vi "Circular Buffer Waveform.vi"(6 "Action":T1, 8 "Error In":errorcluster, 9 "New Data":waveform(dbl), 10 "Size":i32) -> (0 "Error Out":errorcluster, 1 "Buffer Out":waveform(dbl)[](array[waveform]), 2 "Iterations":i32, 5 "Ready":bool)   [LabVIEW 2015]
uses:
  Circular Buffer Operations.ctl
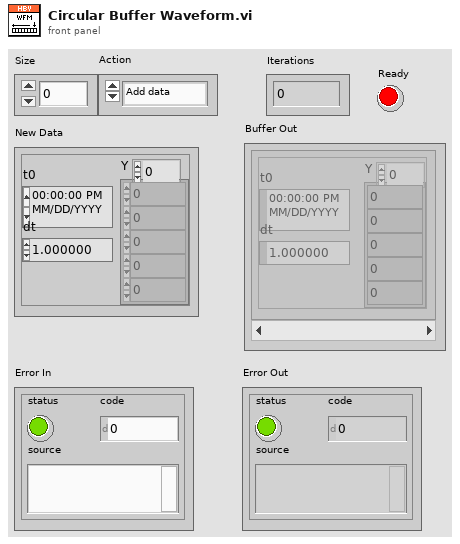
[diagram p1: front panel]
types:
  T1 = typedef "Circular Buffer Operations.ctl" = enum16{"Add data", "Reset"}
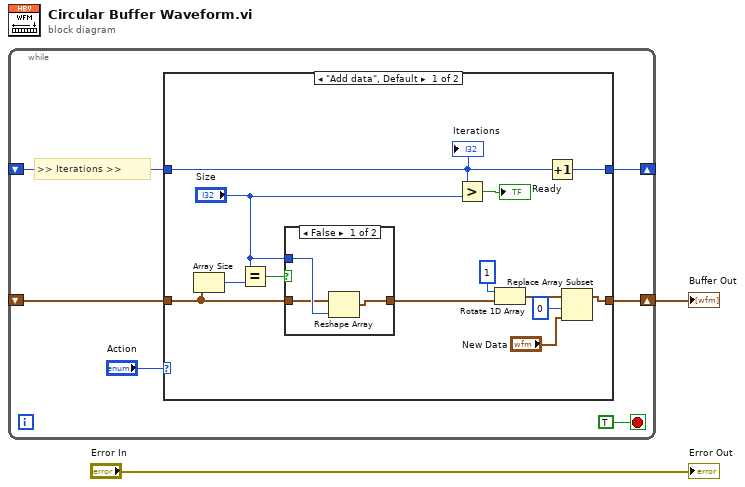
[diagram p0: block diagram]
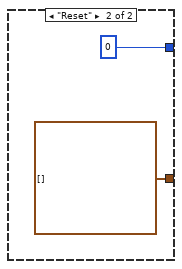
[diagram p3: hidden frame]
diagram:
  n1 = while {
    shift-right: [w8] -> w2
    shift-left: _ -> [w7]
    shift-right: [w4] -> _
    shift-left: _ -> [w3]
    stop <- TRUE stop-if-true
    # ">> Iterations >>"
    n2 = case shown="\"Add data\", Default" "Action" {
      tunnel: [w18 waveform(dbl)[] []] -> w8
      tunnel: w7 -> [w11 _]
      tunnel: [w16 0] -> w4
      tunnel: w3 -> [w15 _]
      frame "Add data", Default {
        n3 = Array Size(array=w11) -> (size(s)=w13:i32)
        n4 = Equal?(x="Size", y=w13) -> (x = y?=w12:bool)
        n5 = case shown="False" w12 {
          tunnel: "Size" -> [w24 _]
          tunnel: w11 -> [w23 w25]
          tunnel: [w22 w25] -> w10
          frame False {
            n6 = Reshape Array(w23, w24) -> (w22:waveform(dbl)[])
          }
          frame True {
          }
        }
        n7 = Greater?(x=w15, y="Size") -> (0:→"Ready":bool)
        n8 = Rotate 1D Array(1:w10, 2:1 ("n")) -> (0:w19:waveform(dbl)[])
        n9 = Increment(x=w15) -> (x+1=w16:i32)
        n10 = Replace Array Subset(array=w19, new element="New Data", index=0) -> (w18:waveform(dbl)[])
        "Iterations" <- w15
      }
      frame "Reset" {
      }
    }
  }
  "Buffer Out" <- w2
  "Error Out" <- "Error In"
